vi "Create Log Queues.vi"(8 "error in (no error)":errorcluster, 11 "Waveform Logs in":T2[](array[typedef]) {"Node ID" format="%.0x"; "TDMS Error Code"."Data Ref" format="%.0x"; "Missed Samples"."Data Ref" format="%.0x"; "File Status"."Data Ref" format="%.0x"; "Start New File"."Data Ref" format="%.0x"; "Logging Enabled"."Data Ref" format="%.0x"; "Stop Trigger"."Node Data Ref" format="%.0x"; "Stop Trigger"."Node ID" format="%.0x"; "Start Trigger"."Node Data Ref" format="%.0x"; "Start Trigger"."Node ID" format="%.0x"}) -> (0 "error out":errorcluster, 2 "Logging Queues":T1[](array[typedef]), 3 "Waveform Logs out":T2[](array[typedef]) {"Node ID" format="%.0x"; "TDMS Error Code"."Data Ref" format="%.0x"; "Missed Samples"."Data Ref" format="%.0x"; "File Status"."Data Ref" format="%.0x"; "Start New File"."Data Ref" format="%.0x"; "Logging Enabled"."Data Ref" format="%.0x"; "Stop Trigger"."Node Data Ref" format="%.0x"; "Stop Trigger"."Node ID" format="%.0x"; "Start Trigger"."Node Data Ref" format="%.0x"; "Start Trigger"."Node ID" format="%.0x"})   [LabVIEW 2015, in "Waveform Data Logger Engine.lvlib"]
uses:
  Waveform Data Logger Engine.lvlib
  Types/Inline Waveform Log Info.ctl
  Shared/Classes/Log File Specifications/Waveform TDMS Log File Specification/Waveform TDMS Log File Specification.lvclass
  Classes/Triggers/Trigger/Trigger.lvclass
  <vilib>/NI Veristand/Custom Device API/Custom Device Item Ref.ctl
  Types/Inline Log Waveform.ctl
  Types/Trigger Settings.ctl
  Types/Log Status.ctl
  Types/Channel.ctl
  <vilib>/NI Veristand/Custom Device API/Data Reference.ctl
  Types/Log Queues.ctl
  <vilib>/NI VeriStand/Custom Device API/Custom Device API.lvlib
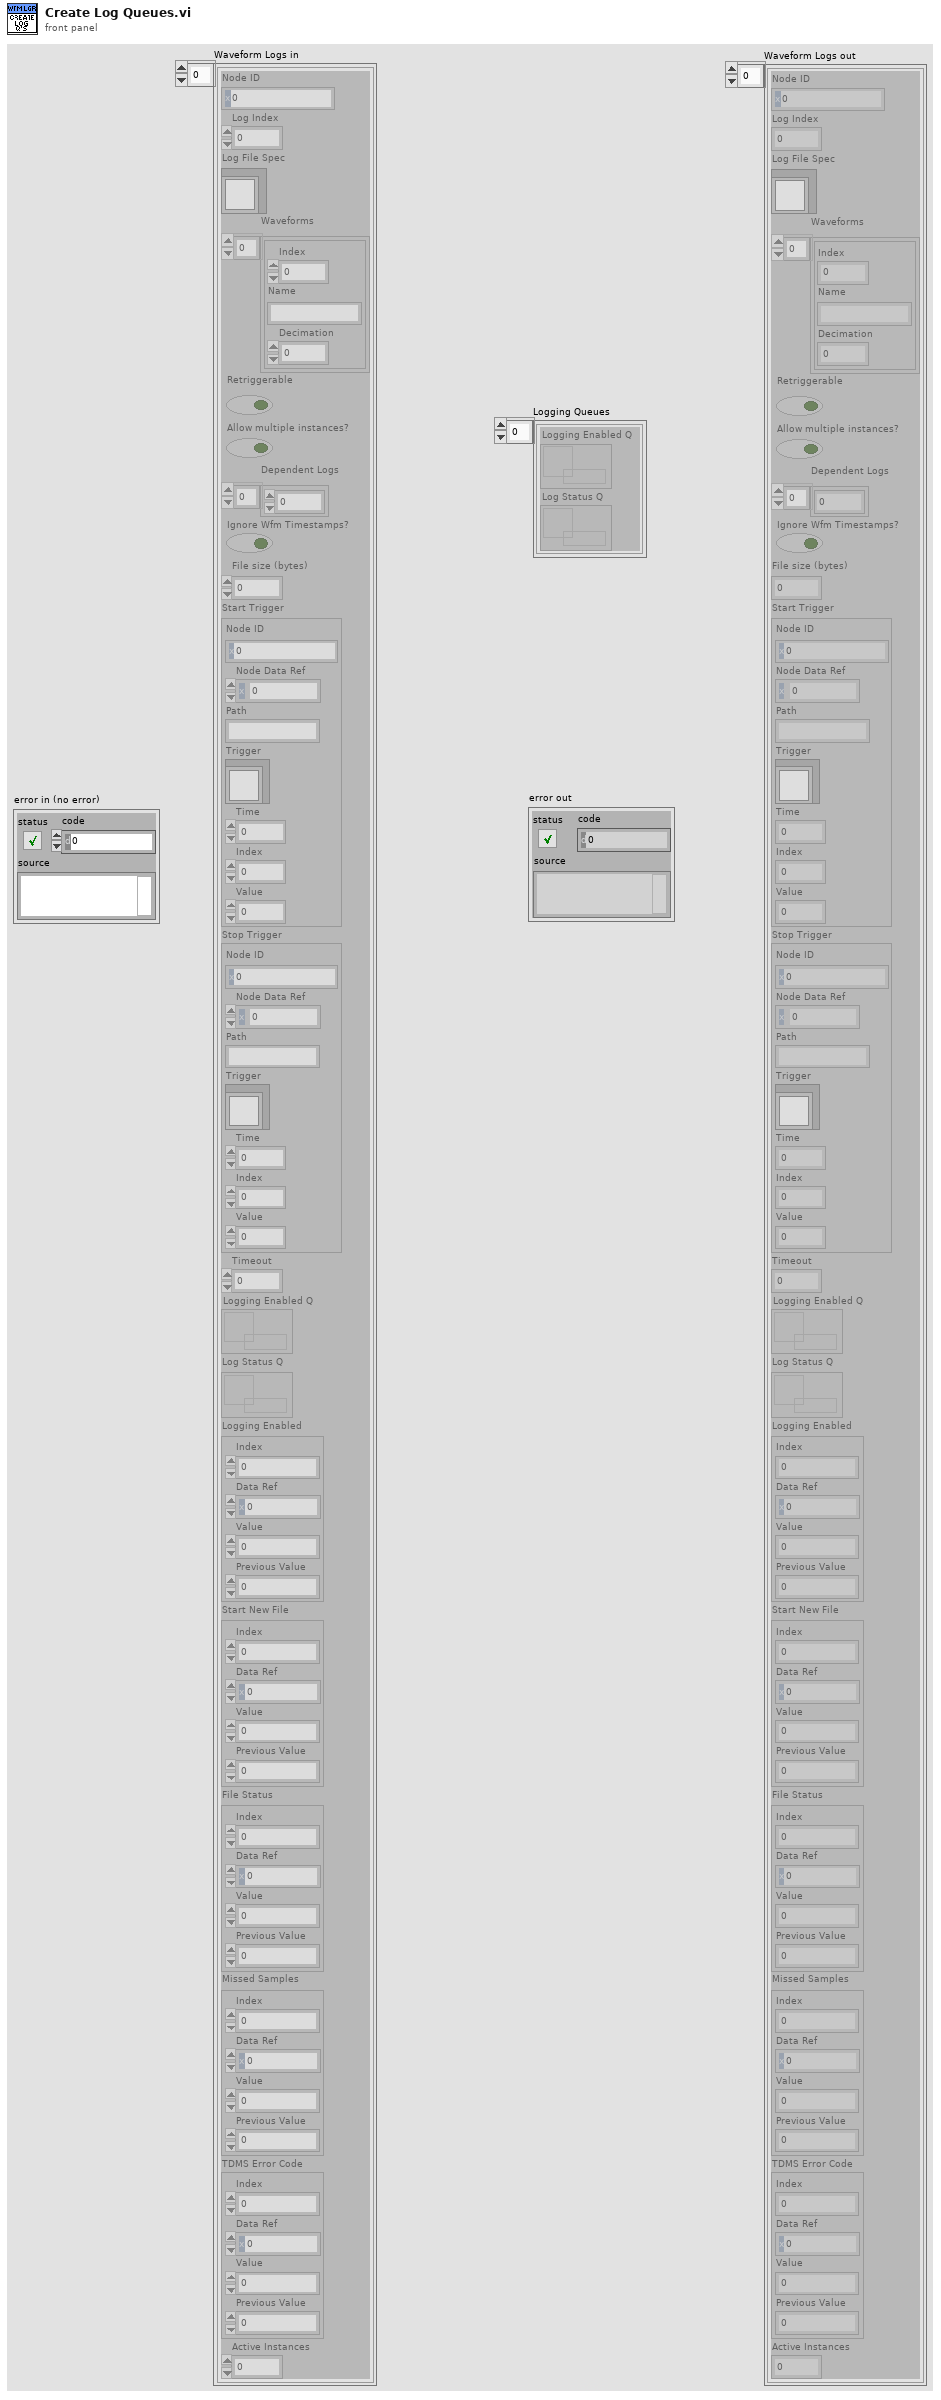
[diagram p1: front panel]
types:
  T1 = typedef "Waveform Data Logger Engine.lvlib/Log Queues.ctl" = cluster{"Logging Enabled Q":refnum<queue>, "Log Status Q":refnum<queue>}
  T2 = typedef "Waveform Data Logger Engine.lvlib/Inline Waveform Log Info.ctl" = cluster{"Node ID":T3, "Log Index":i32, "Log File Spec":refnum<class "Waveform TDMS Log File Specification.lvclass">, "Waveforms":T4[], "Retriggerable":bool, "Allow multiple instances?":bool, "Dependent Logs":i32[], "Ignore Wfm Timestamps?":bool, "File size (bytes)":i64, "Start Trigger":T5, "Stop Trigger":T5, "Timeout":dbl, "Logging Enabled Q":refnum<queue>, "Log Status Q":refnum<queue>, "Logging Enabled":T6, "Start New File":T6, "File Status":T6, "Missed Samples":T6, "TDMS Error Code":T6, "Active Instances":i32}
  T3 = typedef "Custom Device API.lvlib/Custom Device Item Ref.ctl" = u64
  T4 = typedef "Waveform Data Logger Engine.lvlib/Inline Log Waveform.ctl" = cluster{"Index":i32, "Name":string, "Decimation":u32}
  T5 = typedef "Waveform Data Logger Engine.lvlib/Trigger Settings.ctl" = cluster{"Node ID":T3, "Node Data Ref":i32, "Path":string, "Trigger":refnum<class "Trigger.lvclass">, "Time":dbl, "Index":i32, "Value":dbl}
  T6 = typedef "Waveform Data Logger Engine.lvlib/Channel.ctl" = cluster{"Index":i32, "Data Ref":T7, "Value":dbl, "Previous Value":dbl}
  T7 = typedef "Custom Device API.lvlib/Data Reference.ctl" = i32
  T8 = typedef "Waveform Data Logger Engine.lvlib/Log Status.ctl" = cluster{"Open Instances":i32, "Active Instances":i32, "Missed Samples":u64, "Error Code":i32}
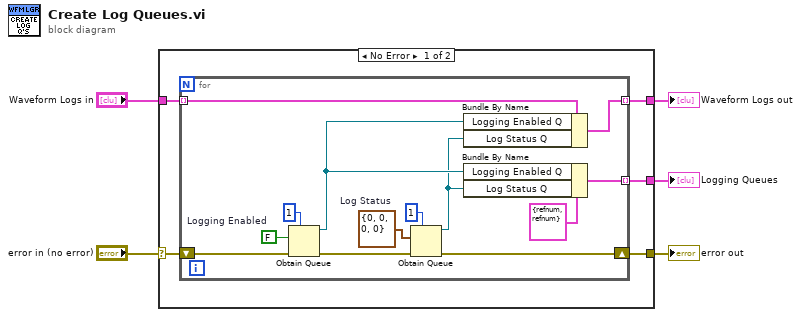
[diagram p0: block diagram]
diagram:
  n1 = case shown="No Error" "error in (no error)" {
    selector: "error in (no error)" -> [w9 w24]
    tunnel: [w7 w24] -> w4
    tunnel: [w8 w25] -> w3
    tunnel: "Waveform Logs in" -> [w10 w25]
    tunnel: [w6 _] -> w1
    frame No Error {
      n2 = for {
        tunnel: w10 -> [w23] mode=indexing
        shift-right: [w15] -> w7
        shift-left: w9 -> [w21]
        tunnel: [w16] -> w8 mode=indexing
        tunnel: [w11] -> w6 mode=indexing
        w17 = FALSE  # Logging Enabled
        w20 = T8 {"Open Instances"=0, "Active Instances"=0, "Missed Samples"=0, "Error Code"=0}  # Log Status
        n3 = Obtain Queue(max queue size (-1, unlimited)=1, element data type=w17, error in (no error)=w21) -> (queue out=w13:refnum<queue>, error out=w18:errorcluster)  [unwired: 2 in, 1 out]
        n4 = Obtain Queue(max queue size (-1, unlimited)=1, element data type=w20, error in (no error)=w18) -> (queue out=w12:refnum<queue>, error out=w15:errorcluster)  [unwired: 2 in, 1 out]
        n5 = Bundle By Name(cluster=w23, "Logging Enabled Q"=w13, "Log Status Q"=w12) -> (w16:T2)
        n6 = Bundle By Name(cluster=T1 {"Logging Enabled Q"=refnum, "Log Status Q"=refnum} ("Log Queues"), "Logging Enabled Q"=w13, "Log Status Q"=w12) -> (w11:T1)
      }
    }
    frame Error {
    }
  }
  "error out" <- w4
  "Waveform Logs out" <- w3
  "Logging Queues" <- w1
